vi "USB_Get_Device_Descriptor_CONFIGURATION.vi"(4 "error out 2":errorcluster, 7 "VISA resource name":refnum<visa-resource-name>) -> (0 "error out":errorcluster, 1 "Interface":T4, 2 "USB_Standard Configuration Descriptor":T5, 3 "VISA resource name 2":refnum<visa-resource-name>)   [LabVIEW 2014]
uses:
  Helper VIs/bmRequestType_recipient.ctl
  Helper VIs/bmRequestType_type.ctl
  Helper VIs/bmRequestType_direction.ctl
  Helper VIs/bmRequestType Parameters.ctl
  Helper VIs/bRequest.ctl
  Standard Descriptor Types/USB_Standard Configuration Descriptor.ctl
  Standard Descriptor Types/USB_Descriptor Type.ctl
  Standard Descriptor Types/USB_Standard Interface Descriptor.ctl
  Standard Descriptor Types/USB_Standard Endpoint Descriptor.ctl
  Standard Descriptor Types/USB_Device Class.ctl
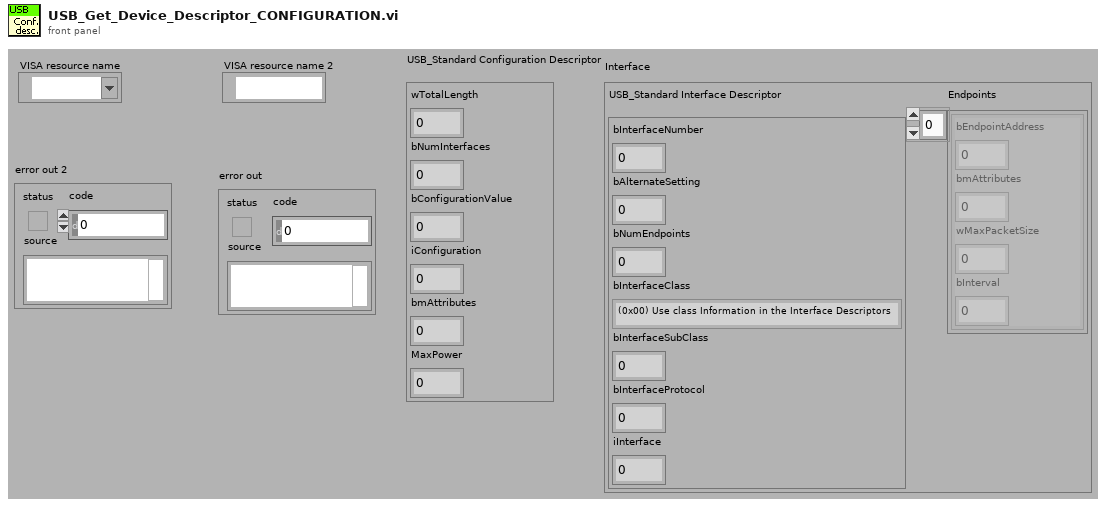
[diagram p1: front panel]
types:
  T1 = typedef "USB_Standard Interface Descriptor.ctl" = cluster{"bInterfaceNumber":u8, "bAlternateSetting":u8, "bNumEndpoints":u8, "bInterfaceClass":T2, "bInterfaceSubClass":u8, "bInterfaceProtocol":u8, "iInterface":u8}
  T2 = typedef "USB_Device Class.ctl" = enum8{"(0x00) Use class Information in the Interface Descriptors", "(0x01) Audio", "(0x02) Communications and CDC Control", "(0x03) HID (Human Interface Device)", "(0x04) Reserved", "(0x05) Physical", "(0x06) Image", "(0x07) Printer", "(0x08) Mass Storage", "(0x09) Hub", "(0x0A) CDC-Data", "(0x0B) Smart Card", "(0x0C) Reserved", "(0x0D) Content Security", "(0x0E) Video", "(0x0F) Personal Healthcare", "(0x10) Reserved", "(0x11) Reserved", "(0x12) Reserved", "(0x13) Reserved", "(0x14) Reserved", "(0x15) Reserved", "(0x16) Reserved", "(0x17) Reserved", "(0x18) Reserved", "(0x19) Reserved", "(0x1A) Reserved", "(0x1B) Reserved", "(0x1C) Reserved", "(0x1D) Reserved", "(0x1E) Reserved", "(0x1F) Reserved", "(0x20) Reserved", "(0x21) Reserved", "(0x22) Reserved", "(0x23) Reserved", "(0x24) Reserved", "(0x25) Reserved", "(0x26) Reserved", "(0x27) Reserved", "(0x28) Reserved", "(0x29) Reserved", "(0x2A) Reserved", "(0x2B) Reserved", "(0x2C) Reserved", "(0x2D) Reserved", "(0x2E) Reserved", "(0x2F) Reserved", "(0x30) Reserved", "(0x31) Reserved", "(0x32) Reserved", "(0x33) Reserved", "(0x34) Reserved", "(0x35) Reserved", "(0x36) Reserved", "(0x37) Reserved", "(0x38) Reserved", "(0x39) Reserved", "(0x3A) Reserved", "(0x3B) Reserved", "(0x3C) Reserved", "(0x3D) Reserved", "(0x3E) Reserved", "(0x3F) Reserved", "(0x40) Reserved", "(0x41) Reserved", "(0x42) Reserved", "(0x43) Reserved", "(0x44) Reserved", "(0x45) Reserved", "(0x46) Reserved", "(0x47) Reserved", "(0x48) Reserved", "(0x49) Reserved", "(0x4A) Reserved", "(0x4B) Reserved", "(0x4C) Reserved", "(0x4D) Reserved", "(0x4E) Reserved", "(0x4F) Reserved", "(0x50) Reserved", "(0x51) Reserved", "(0x52) Reserved", "(0x53) Reserved", "(0x54) Reserved", "(0x55) Reserved", "(0x56) Reserved", "(0x57) Reserved", "(0x58) Reserved", "(0x59) Reserved", "(0x5A) Reserved", "(0x5B) Reserved", "(0x5C) Reserved", "(0x5D) Reserved", "(0x5E) Reserved", "(0x5F) Reserved", "(0x60) Reserved", "(0x61) Reserved", "(0x62) Reserved", "(0x63) Reserved", "(0x64) Reserved", "(0x65) Reserved", "(0x66) Reserved", "(0x67) Reserved", "(0x68) Reserved", "(0x69) Reserved", "(0x6A) Reserved", "(0x6B) Reserved", "(0x6C) Reserved", "(0x6D) Reserved", "(0x6E) Reserved", "(0x6F) Reserved", "(0x70) Reserved", "(0x71) Reserved", "(0x72) Reserved", "(0x73) Reserved", "(0x74) Reserved", "(0x75) Reserved", "(0x76) Reserved", "(0x77) Reserved", "(0x78) Reserved", "(0x79) Reserved", "(0x7A) Reserved", "(0x7B) Reserved", "(0x7C) Reserved", "(0x7D) Reserved", "(0x7E) Reserved", "(0x7F) Reserved", "(0x80) Reserved", "(0x81) Reserved", "(0x82) Reserved", "(0x83) Reserved", "(0x84) Reserved", "(0x85) Reserved", "(0x86) Reserved", "(0x87) Reserved", "(0x88) Reserved", "(0x89) Reserved", "(0x8A) Reserved", "(0x8B) Reserved", "(0x8C) Reserved", "(0x8D) Reserved", "(0x8E) Reserved", "(0x8F) Reserved", "(0x90) Reserved", "(0x91) Reserved", "(0x92) Reserved", "(0x93) Reserved", "(0x94) Reserved", "(0x95) Reserved", "(0x96) Reserved", "(0x97) Reserved", "(0x98) Reserved", "(0x99) Reserved", "(0x9A) Reserved", "(0x9B) Reserved", "(0x9C) Reserved", "(0x9D) Reserved", "(0x9E) Reserved", "(0x9F) Reserved", "(0xA0) Reserved", "(0xA1) Reserved", "(0xA2) Reserved", "(0xA3) Reserved", "(0xA4) Reserved", "(0xA5) Reserved", "(0xA6) Reserved", "(0xA7) Reserved", "(0xA8) Reserved", "(0xA9) Reserved", "(0xAA) Reserved", "(0xAB) Reserved", "(0xAC) Reserved", "(0xAD) Reserved", "(0xAE) Reserved", "(0xAF) Reserved", "(0xB0) Reserved", "(0xB1) Reserved", "(0xB2) Reserved", "(0xB3) Reserved", "(0xB4) Reserved", "(0xB5) Reserved", "(0xB6) Reserved", "(0xB7) Reserved", "(0xB8) Reserved", "(0xB9) Reserved", "(0xBA) Reserved", "(0xBB) Reserved", "(0xBC) Reserved", "(0xBD) Reserved", "(0xBE) Reserved", "(0xBF) Reserved", "(0xC0) Reserved", "(0xC1) Reserved", "(0xC2) Reserved", "(0xC3) Reserved", "(0xC4) Reserved", "(0xC5) Reserved", "(0xC6) Reserved", "(0xC7) Reserved", "(0xC8) Reserved", "(0xC9) Reserved", "(0xCA) Reserved", "(0xCB) Reserved", "(0xCC) Reserved", "(0xCD) Reserved", "(0xCE) Reserved", "(0xCF) Reserved", "(0xD0) Reserved", "(0xD1) Reserved", "(0xD2) Reserved", "(0xD3) Reserved", "(0xD4) Reserved", "(0xD5) Reserved", "(0xD6) Reserved", "(0xD7) Reserved", "(0xD8) Reserved", "(0xD9) Reserved", "(0xDA) Reserved", "(0xDB) Reserved", "(0xDC) Reserved", "(0xDD) Reserved", "(0xDE) Reserved", "(0xDF) Reserved", "(0xE0) Reserved", "(0xE1) Reserved", "(0xE2) Reserved", "(0xE3) Reserved", "(0xE4) Reserved", "(0xE5) Reserved", "(0xE6) Reserved", "(0xE7) Reserved", "(0xE8) Reserved", "(0xE9) Reserved", "(0xEA) Reserved", "(0xEB) Reserved", "(0xEC) Reserved", "(0xED) Reserved", "(0xEE) Reserved", "(0xEF) Reserved", "(0xF0) Reserved", "(0xF1) Reserved", "(0xF2) Reserved", "(0xF3) Reserved", "(0xF4) Reserved", "(0xF5) Reserved", "(0xF6) Reserved", "(0xF7) Reserved", "(0xF8) Reserved", "(0xF9) Reserved", "(0xFA) Reserved", "(0xFB) Reserved", "(0xFC) Reserved", "(0xFD) Reserved", "(0xFE) Reserved", "(0xFF) Reserved"}
  T3 = typedef "USB_Standard Endpoint Descriptor.ctl" = cluster{"bEndpointAddress":u8, "bmAttributes":u8, "wMaxPacketSize":u16, "bInterval":u8}
  T4 = cluster{"USB_Standard Interface Descriptor":T1, "Endpoints":T3[]}
  T5 = typedef "USB_Standard Configuration Descriptor.ctl" = cluster{"wTotalLength":u16, "bNumInterfaces":u8, "bConfigurationValue":u8, "iConfiguration":u8, "bmAttributes":u8, "MaxPower":u8}
  T6 = typedef "bRequest.ctl" = enum8{"GET_STATUS", "CLEAR_FEATURE", "Reserved (2)", "SET_FEATURE", "Reserved (4)", "SET_ADDRESS", "GET_DESCRIPTOR", "SET_DESCRIPTOR", "GET_CONFIGURATION", "SET_CONFIGURATION", "GET_INTERFACE", "SET_INTERFACE", "SYNCH_FRAME", "<OTHER>"}
  T7 = typedef "bmRequestType Parameters.ctl" = cluster{"Direction":T8, "Type":T9, "Recipient":T10}
  T8 = typedef "bmRequestType_direction.ctl" = enum16{"Host-to-Device", "Device-to-Host"}
  T9 = typedef "bmRequestType_type.ctl" = enum16{"Standard", "Class", "Vendor"}
  T10 = typedef "bmRequestType_recipient.ctl" = enum16{"Device", "Interface", "Endpoint", "Other"}
  T11 = typedef "USB_Descriptor Type.ctl" = enum8{"INVALID", "DEVICE (0x01)", "CONFIGURATION (0x02)", "STRING (0x03)", "INTERFACE (0x04)", "ENDPOINT (0x05)", "DEVICE_QUALIFIER (0x06)", "OTHER_SPEED_CONFIGURATION (0x07)", "INTERFACE_POWER (0x08)", "OTG (0x09)", "DEBUG (0x0A)", "INTERFACE ASSOCIATION (0x0B)", "Unknown (0x0C)", "Unknown (0x0D)", "Unknown (0x0E)", "Unknown (0x0F)", "Unknown (0x10)", "Unknown (0x11)", "Unknown (0x12)", "Unknown (0x13)", "Unknown (0x14)", "Unknown (0x15)", "Unknown (0x16)", "Unknown (0x17)", "Unknown (0x18)", "Unknown (0x19)", "Unknown (0x1A)", "Unknown (0x1B)", "Unknown (0x1C)", "Unknown (0x1D)", "Unknown (0x1E)", "Unknown (0x1F)", "Unknown (0x20)", "HID (0x21)", "HID Report (0x22)", "HID Physical Decriptor (0x23)", "HID Reserved (0x24)", "HID Reserved (0x25)", "HID Reserved (0x26)", "HID Reserved (0x27)", "HID Reserved (0x28)", "HID Reserved (0x29)", "HID Reserved (0x2A)", "HID Reserved (0x2B)", "HID Reserved (0x2C)", "HID Reserved (0x2D)", "HID Reserved (0x2E)", "HID Reserved (0x2F)"}
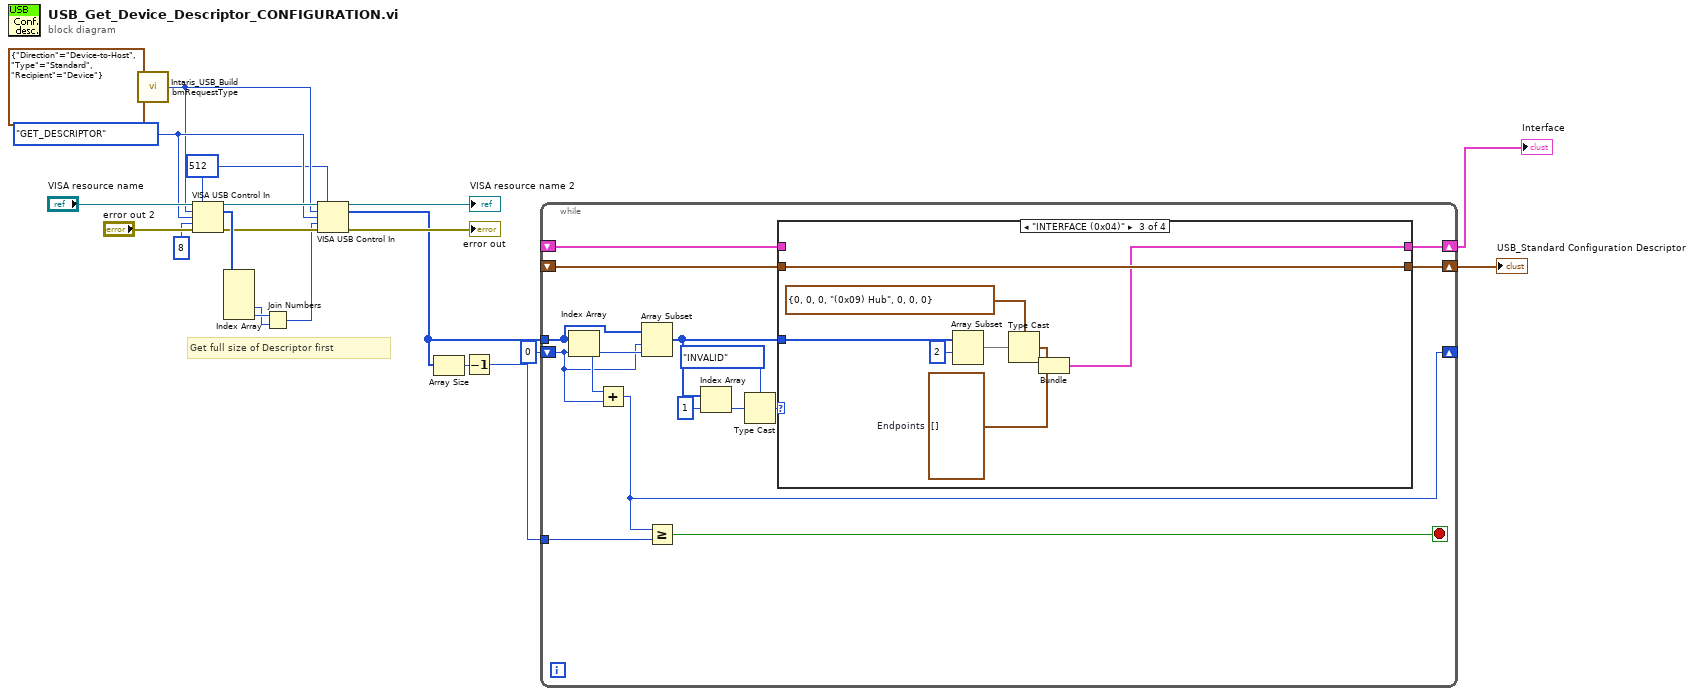
[diagram p0: block diagram]
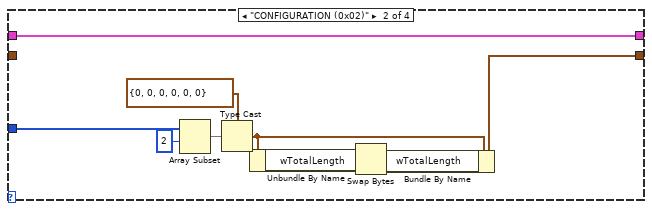
[diagram p3: hidden frame]
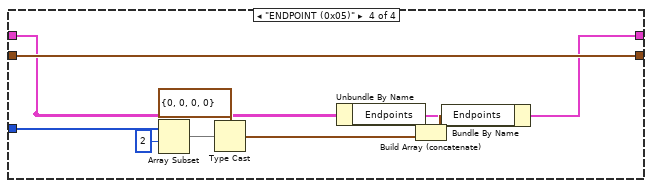
[diagram p4: hidden frame]
diagram:
  w4 = bRequest."GET_DESCRIPTOR" ("bRequest")
  w2 = u16 512
  # "Get full size of Descriptor first"
  n1 = call "Intaris_USB_Build bmRequestType.vi"("bmRequest Parameters"=T7 {"Direction"=enum."Device-to-Host", "Type"=enum."Standard", "Recipient"=enum."Device"}) -> ("bmRequest"=w3:i16)  [unwired: 4 in]
  n2 = VISA USB Control In(0:"VISA resource name", 1:w2, 5:w3, 7:w4, 9:u16 8 ("length (0)"), 11:"error out 2") -> (4:w9:refnum<visa-resource-name>, 6:w12:u8[], 15:w8:errorcluster)  [unwired: 1 in]
  n3 = Index Array(array=w12) -> (element #3=w10:u8, element #4=w11:u8)  [unwired: 4 in, 2 out]
  n4 = Join Numbers(hi=w11, lo=w10) -> ((hi.lo)=w5:u16)
  n5 = VISA USB Control In(0:w9, 1:w2, 5:w3, 7:w4, 9:w5, 11:w8) -> (4:→"VISA resource name 2":refnum<visa-resource-name>, 6:w1:u8[], 15:→"error out":errorcluster)  [unwired: 1 in]
  n6 = Array Size(array=w1) -> (size(s)=w16:i32)
  n7 = Decrement(x=w16) -> (x-1=w15:i32)
  n8 = while {
    shift-right: [w29] -> _
    shift-left: 0 -> [w26]
    tunnel: w1 -> [w36]
    tunnel: w15 -> [w28]
    shift-right: [w25] -> w14
    shift-left: _ -> [w24]
    shift-right: [w22] -> w13
    shift-left: _ -> [w23]
    stop <- w27 stop-if-true
    n9 = Index Array(array=w36, index=w26) -> (element=w30:u8)
    n10 = Add(x=w30, y=w26) -> (x+y=w29:i32)
    n11 = Array Subset(array=w36, index=w26, length=w30) -> (w31:u8[])
    n12 = Greater Or Equal?(x=w29, y=w28) -> (x >= y?=w27:bool)
    n13 = Index Array(array=w31, index=1) -> (element=w33:u8)
    n14 = Type Cast(type=USB_Descriptor_Type."INVALID" ("bDescriptorType"), x=w33) -> (*(type *) &x=w32:T11)
    n15 = case shown="\"INTERFACE (0x04)\"" w32 {
      tunnel: w31 -> [_ w45 w51 w61]
      tunnel: [w38 w40 w55 w65] -> w25
      tunnel: w24 -> [w38 _ w55 w65]
      tunnel: w23 -> [w37 w39 _ w57]
      tunnel: [w37 w39 w48 w56] -> w22
      frame "INVALID", Default {
      }
      frame "CONFIGURATION (0x02)" {
        n16 = Array Subset(array=w45, index=2) -> (w44:u8[])  [unwired: 1 in]
        n17 = Type Cast(type=T5 {"wTotalLength"=0, "bNumInterfaces"=0, "bConfigurationValue"=0, "iConfiguration"=0, "bmAttributes"=0, "MaxPower"=0} ("USB_Standard Configuration Descriptor"), x=w44) -> (*(type *) &x=w42:T5)
        n18 = Unbundle By Name(w42) -> ("wTotalLength"=w43:u16)
        n19 = Swap Bytes(anything=w43) -> (byte swapped=w41:u16)
        n20 = Bundle By Name(cluster=w42, "wTotalLength"=w41) -> (w40:T5)
      }
      frame "INTERFACE (0x04)" {
        w49 = T3[] []  # Endpoints
        n21 = Array Subset(array=w51, index=2) -> (w53:u8[])  [unwired: 1 in]
        n22 = Type Cast(type=T1 {"bInterfaceNumber"=0, "bAlternateSetting"=0, "bNumEndpoints"=0, "bInterfaceClass"=enum."(0x09) Hub", "bInterfaceSubClass"=0, "bInterfaceProtocol"=0, "iInterface"=0} ("USB_Standard Interface Descriptor"), x=w53) -> (*(type *) &x=w50:T1)
        n23 = Bundle("USB_Standard Interface Descriptor"=w50, "Endpoints"=w49) -> (w48:T4)  [unwired: 1 in]
      }
      frame "ENDPOINT (0x05)" {
        n24 = Array Subset(array=w61, index=2) -> (w63:u8[])  [unwired: 1 in]
        n25 = Type Cast(type=T3 {"bEndpointAddress"=0, "bmAttributes"=0, "wMaxPacketSize"=0, "bInterval"=0} ("USB_Standard Endpoint Descriptor"), x=w63) -> (*(type *) &x=w59:T3)
        n26 = Unbundle By Name(w57) -> ("Endpoints"=w60:T3[])
        n27 = Build Array (concatenate)(w60, w59) -> (w58:T3[])
        n28 = Bundle By Name(cluster=w57, "Endpoints"=w58) -> (w56:T4)
      }
    }
  }
  "USB_Standard Configuration Descriptor" <- w14
  "Interface" <- w13
